vi "OscAutoDiap (SubVI).vi"(9 "Numeric":i16, 10 "MaxADCvalue":i16, 11 "Range":u16) -> (3 "y":i16)   [LabVIEW 2017]
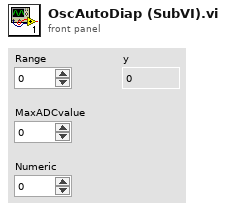
[diagram p1: front panel]
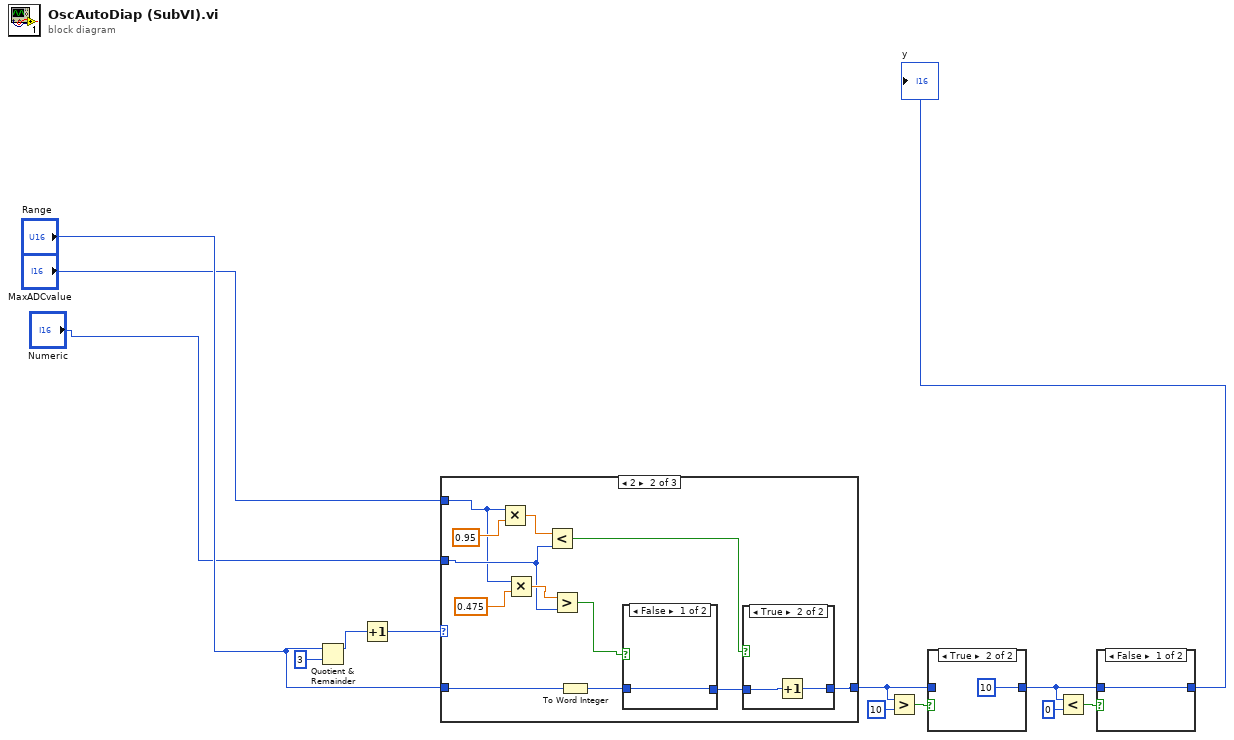
[diagram p0: block diagram]
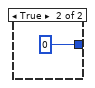
[diagram p2: hidden frame]
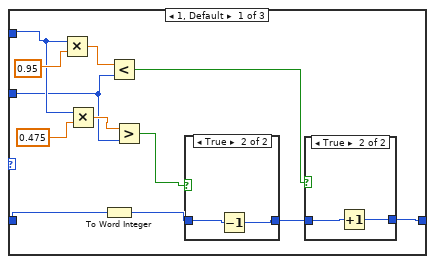
[diagram p4: hidden frame]
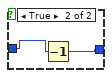
[diagram p7: hidden frame]
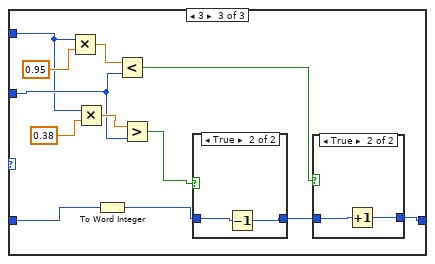
[diagram p9: hidden frame]
diagram:
  n1 = Quotient & Remainder(x="Range", y=u16 3) -> (x-y*floor(x/y)=w2:u16)  [unwired: 1 out]
  n2 = Increment(x=w2) -> (x+1=w3:u16)
  n3 = case shown="2" w3 {
    tunnel: "Numeric" -> [w17 w36 w53]
    tunnel: "Range" -> [w14 w32 w50]
    tunnel: [w22 w34 w54] -> w5
    tunnel: "MaxADCvalue" -> [w19 w35 w52]
    frame 1, Default {
      n4 = Multiply(x=w19, y=0.95) -> (x*y=w24:dbl)
      n5 = Multiply(x=w19, y=0.475) -> (x*y=w18:dbl)
      n6 = To Word Integer(number=w14) -> (16bit integer=w15:i16)
      n7 = Less?(x=w24, y=w17) -> (x < y?=w23:bool)
      n8 = Greater?(x=w18, y=w17) -> (0:w16:bool)
      n9 = case shown="True" w16 {
        tunnel: w15 -> [w26 w27]
        tunnel: [w26 w28] -> w21
        frame False {
        }
        frame True {
          n10 = Decrement(x=w27) -> (x-1=w28:i16)
        }
      }
      n11 = case shown="True" w23 {
        tunnel: w21 -> [w29 w30]
        tunnel: [w29 w31] -> w22
        frame False {
        }
        frame True {
          n12 = Increment(x=w30) -> (x+1=w31:i16)
        }
      }
    }
    frame 2 {
      n13 = Multiply(x=w35, y=0.95) -> (x*y=w42:dbl)
      n14 = Multiply(x=w35, y=0.475) -> (x*y=w38:dbl)
      n15 = Less?(x=w42, y=w36) -> (x < y?=w41:bool)
      n16 = Greater?(x=w38, y=w36) -> (0:w37:bool)
      n17 = To Word Integer(number=w32) -> (16bit integer=w33:i16)
      n18 = case shown="False" w37 {
        tunnel: [w44 w46] -> w40
        tunnel: w33 -> [w44 w45]
        frame False {
        }
        frame True {
          n19 = Decrement(x=w45) -> (x-1=w46:i16)
        }
      }
      n20 = case shown="True" w41 {
        tunnel: w40 -> [w47 w48]
        tunnel: [w47 w49] -> w34
        frame False {
        }
        frame True {
          n21 = Increment(x=w48) -> (x+1=w49:i16)
        }
      }
    }
    frame 3 {
      n22 = Multiply(x=w52, y=0.95) -> (x*y=w60:dbl)
      n23 = Multiply(x=w52, y=0.38) -> (x*y=w56:dbl)
      n24 = To Word Integer(number=w50) -> (16bit integer=w51:i16)
      n25 = Less?(x=w60, y=w53) -> (x < y?=w59:bool)
      n26 = Greater?(x=w56, y=w53) -> (0:w55:bool)
      n27 = case shown="True" w55 {
        tunnel: w51 -> [w62 w63]
        tunnel: [w62 w64] -> w58
        frame False {
        }
        frame True {
          n28 = Decrement(x=w63) -> (x-1=w64:i16)
        }
      }
      n29 = case shown="True" w59 {
        tunnel: w58 -> [w65 w66]
        tunnel: [w65 w67] -> w54
        frame False {
        }
        frame True {
          n30 = Increment(x=w66) -> (x+1=w67:i16)
        }
      }
    }
  }
  n31 = Greater?(x=w5, y=i16 10) -> (0:w4:bool)
  n32 = case shown="True" w4 {
    tunnel: w5 -> [w68 _]
    tunnel: [w68 i16 10 ("y")] -> w9
    frame False {
    }
    frame True {
    }
  }
  n33 = Less?(x=w9, y=i16 0) -> (x < y?=w6:bool)
  n34 = case shown="False" w6 {
    tunnel: w9 -> [w70 _]
    tunnel: [w70 i16 0 ("y")] -> w13
    frame False {
    }
    frame True {
    }
  }
  "y" <- w13
